vi "Build Event Log Path.vi"(8 "error in (no error)":errorcluster, 11 "Text File Sink in":refnum<class "Text File Sink.lvclass">) -> (0 "error out":errorcluster, 3 "Text File Sink out":refnum<class "Text File Sink.lvclass">)   [LabVIEW 2017, in "Text File Sink.lvclass"]
doc: "--\nCopyright © 2017 Composed SystemsI All rights reserved.\n\nAuthor: Jon McBee <jon.mcbee@composed.io>\n\nThis library is provided \"AS IS\" ,WITHOUT WARRANTIES OR\nCONDITIONS OF ANY KIND, either express or implied.\n\nComposed Systems -- composed.io\n\nStream 0.0.1.1\nJon McBee - Composed Systems\nCopyright (c) 2017, Composed Systems"
uses:
  <vilib>/gpm_packages/@cs/event-logger/Source/Text File Sink/Text File Sink.lvclass
  <vilib>/gpm_packages/@cs/event-logger/Source/Text File Sink/Text File Sink.lvclass/Text File Sink.ctl
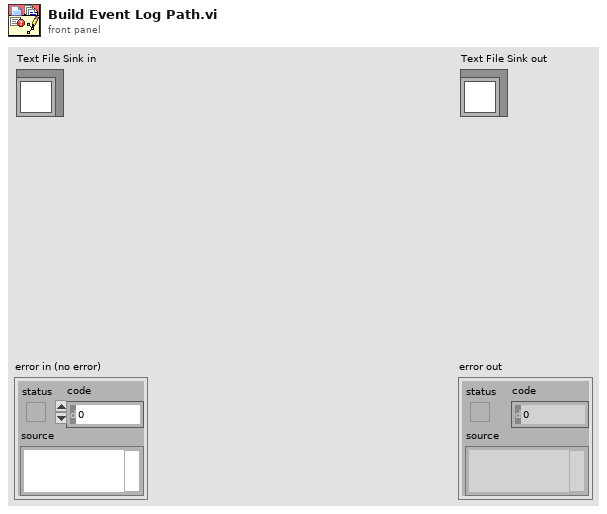
[diagram p1: front panel]
types:
  T1 = typedef "LVDateTimeRec.ctl" = cluster{"fractional second":dbl, "second":i32, "minute":i32, "hour":i32, "day of month":i32, "month":i32, "year":i32, "day of week":i32, "day of year":i32, "DST":i32}
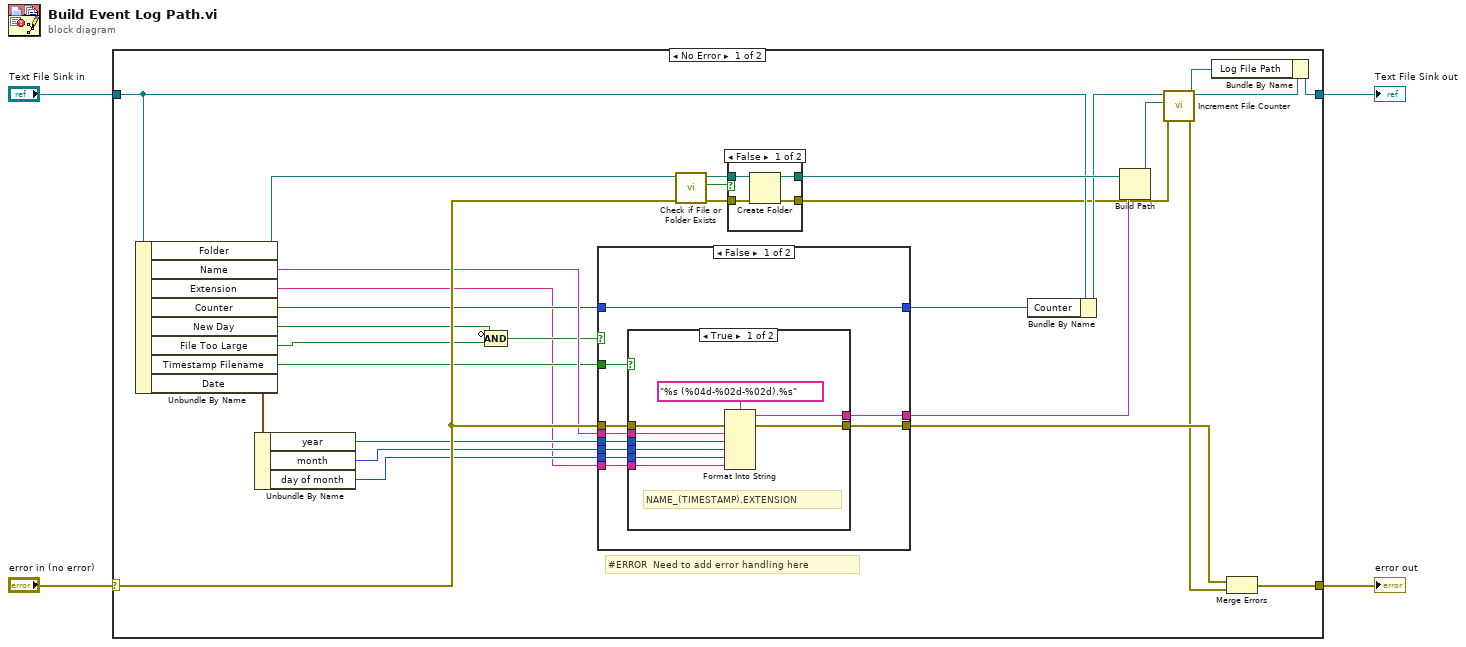
[diagram p0: block diagram]
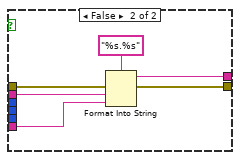
[diagram p3: hidden frame]
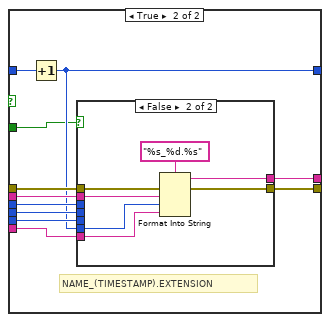
[diagram p4: hidden frame]
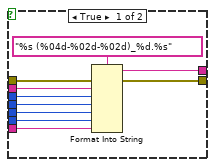
[diagram p5: hidden frame]
diagram:
  n1 = case shown="No Error" "error in (no error)" {
    selector: "error in (no error)" -> [w30 w94]
    tunnel: [w9 w94] -> w3
    tunnel: [w20 w93] -> w1
    tunnel: "Text File Sink in" -> [w19 w93]
    frame No Error {
      # "#ERROR  Need to add error handling here"
      n2 = Unbundle By Name(w19) -> ("Folder"=w31:path, "Name"=w28:string, "Extension"=w8:string, "Counter"=w24:u16, "New Day"=w22:bool, "File Too Large"=w23:bool, "Timestamp Filename"=w12:bool, "Date"=w29:T1)
      n3 = Unbundle By Name(w29) -> ("year"=w27:i32, "month"=w26:i32, "day of month"=w25:i32)
      n4 = Compound Arithmetic op=AND(invert w22, w23) -> (w21:bool)
      n5 = case shown="False" w21 {
        tunnel: [w49 w75] -> w32
        tunnel: [w48 w74] -> w11
        tunnel: w30 -> [w47 w73]
        tunnel: w28 -> [w46 w72]
        tunnel: w27 -> [w45 w71]
        tunnel: w26 -> [w44 w70]
        tunnel: w25 -> [w43 w69]
        tunnel: w8 -> [w42 w68]
        tunnel: w24 -> [w41 w67]
        tunnel: [w41 w66] -> w18
        tunnel: w12 -> [w40 w65]
        frame False {
          n6 = case shown="True" w40 {
            tunnel: [w57 w63] -> w49
            tunnel: [w56 w62] -> w48
            tunnel: w47 -> [w55 w61]
            tunnel: w46 -> [w54 w60]
            tunnel: w45 -> [w53 _]
            tunnel: w44 -> [w52 _]
            tunnel: w43 -> [w51 _]
            tunnel: w42 -> [w50 w59]
            frame True {
              # "NAME_(TIMESTAMP).EXTENSION"
              n7 = Format Into String(format string="%s (%04d-%02d-%02d).%s", error in=w55, w54, w53, w52, w51, w50) -> (resulting string=w57:string, error out=w56:errorcluster)  [unwired: 1 in]
            }
            frame False {
              n8 = Format Into String(format string="%s.%s", error in=w61, w60, w59) -> (resulting string=w63:string, error out=w62:errorcluster)  [unwired: 1 in]
            }
          }
        }
        frame True {
          # "NAME_(TIMESTAMP).EXTENSION"
          n9 = Increment(x=w67) -> (x+1=w66:u16)
          n10 = case shown="False" w65 {
            tunnel: [w84 w91] -> w75
            tunnel: [w83 w90] -> w74
            tunnel: w73 -> [w82 w89]
            tunnel: w72 -> [w81 w88]
            tunnel: w71 -> [w80 _]
            tunnel: w70 -> [w79 _]
            tunnel: w69 -> [w78 _]
            tunnel: w68 -> [w77 w86]
            tunnel: w66 -> [w76 w87]
            frame True {
              n11 = Format Into String(format string="%s (%04d-%02d-%02d)_%d.%s", error in=w82, w81, w80, w79, w78, w76, w77) -> (resulting string=w84:string, error out=w83:errorcluster)  [unwired: 1 in]
            }
            frame False {
              n12 = Format Into String(format string="%s_%d.%s", error in=w89, w88, w87, w86) -> (resulting string=w91:string, error out=w90:errorcluster)  [unwired: 1 in]
            }
          }
        }
      }
      n13 = call <vilib>:"Check if File or Folder Exists.vi"("error in (no error)"=w30, "path"=w31) -> ("error out"=w5:errorcluster, "file or folder exists?"=w7:bool, "dup path"=w6:path)  [unwired: 7 out]
      n14 = case shown="False" w7 {
        tunnel: w6 -> [w36 w39]
        tunnel: w5 -> [w37 w38]
        tunnel: [w35 w38] -> w13
        tunnel: [w34 w39] -> w33
        frame False {
          n15 = Create Folder(path (use dialog)=w36, error in=w37) -> (created path=w34:path, error out=w35:errorcluster)  [unwired: 2 out]
        }
        frame True {
        }
      }
      n16 = Bundle By Name(cluster=w19, "Counter"=w18) -> (w17:refnum<class "Text File Sink.lvclass">)
      n17 = Build Path(base path=w33, name or relative path=w32) -> (appended path=w15:path)
      n18 = call <vilib>:"Increment File Counter.vi"("error in (no error)"=w13, "File Path"=w15, "Text File Sink in"=w17) -> ("error out"=w10:errorcluster, "File Path out"=w14:path, "Text File Sink out"=w16:refnum<class "Text File Sink.lvclass">)  [unwired: 6 in]
      n19 = Bundle By Name(cluster=w16, "Log File Path"=w14) -> (w20:refnum<class "Text File Sink.lvclass">)
      n20 = Merge Errors(w11, w10) -> (w9:errorcluster)
    }
    frame Error {
    }
  }
  "error out" <- w3
  "Text File Sink out" <- w1
